vi "Number-to-two_ASCII_char.vi"(9 "two_byte_num":u32) -> (3 "two_ascii_string":string)   [LabVIEW 2014]
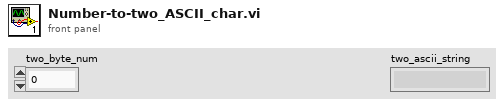
[diagram p1: front panel]
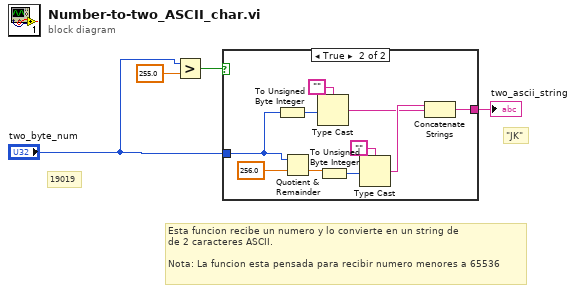
[diagram p0: block diagram]
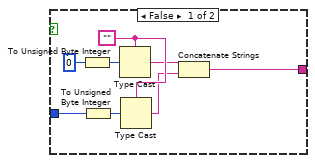
[diagram p2: hidden frame]
diagram:
  # "19019"
  # "\"JK\""
  # "Esta funcion recibe un numero y lo convierte en un string de\nde 2 caracteres ASCII.\n\nNota: La funcion esta pensada para recibir numero menores a 65536"
  n1 = Greater?(x="two_byte_num", y=255.0) -> (0:w1:bool)
  n2 = case shown="True" w1 {
    tunnel: "two_byte_num" -> [w9 w20]
    tunnel: [w5 w15] -> w4
    frame False {
      w8 = ""
      n3 = To Unsigned Byte Integer(number=0) -> (unsigned 8bit integer=w12:u8)
      n4 = To Unsigned Byte Integer(number=w9) -> (unsigned 8bit integer=w10:u8)
      n5 = Type Cast(type=w8, x=w12) -> (*(type *) &x=w7:string)
      n6 = Type Cast(type=w8, x=w10) -> (*(type *) &x=w6:string)
      n7 = Concatenate Strings(w7, w6) -> (w5:string)
    }
    frame True {
      n8 = To Unsigned Byte Integer(number=w20) -> (unsigned 8bit integer=w22:u8)
      n9 = Quotient & Remainder(x=w20, y=256.0) -> (floor(x/y)=w17:dbl)  [unwired: 1 out]
      n10 = Type Cast(type="", x=w22) -> (*(type *) &x=w13:string)
      n11 = To Unsigned Byte Integer(number=w17) -> (unsigned 8bit integer=w18:u8)
      n12 = Type Cast(type="", x=w18) -> (*(type *) &x=w14:string)
      n13 = Concatenate Strings(w14, w13) -> (w15:string)
    }
  }
  "two_ascii_string" <- w4
